vi "AIT 664 - Read Parameters Input VL.vi"(0 "Input VL Parameter File":T1, 5 "Found VL?":bool, 7 "Input VLs":T1[](array[typedef]), 9 "Input VL Configuration File":T1, 11 "error in (no error)":errorcluster) -> (4 "Input VLs out":T1[](array[typedef]), 15 "error out":errorcluster)   [LabVIEW 2013, in "AIT 664 Custom Device.lvlib"]
doc: "Match the parameter file with the configuration file input vls"
uses:
  AIT 664 Custom Device.lvlib
  Controls/664 - XML Input VL.ctl
  Controls/664 - XML Rx Message Port.ctl
  Controls/664 - Sampling Type.ctl
  Controls/664 -Param.ctl
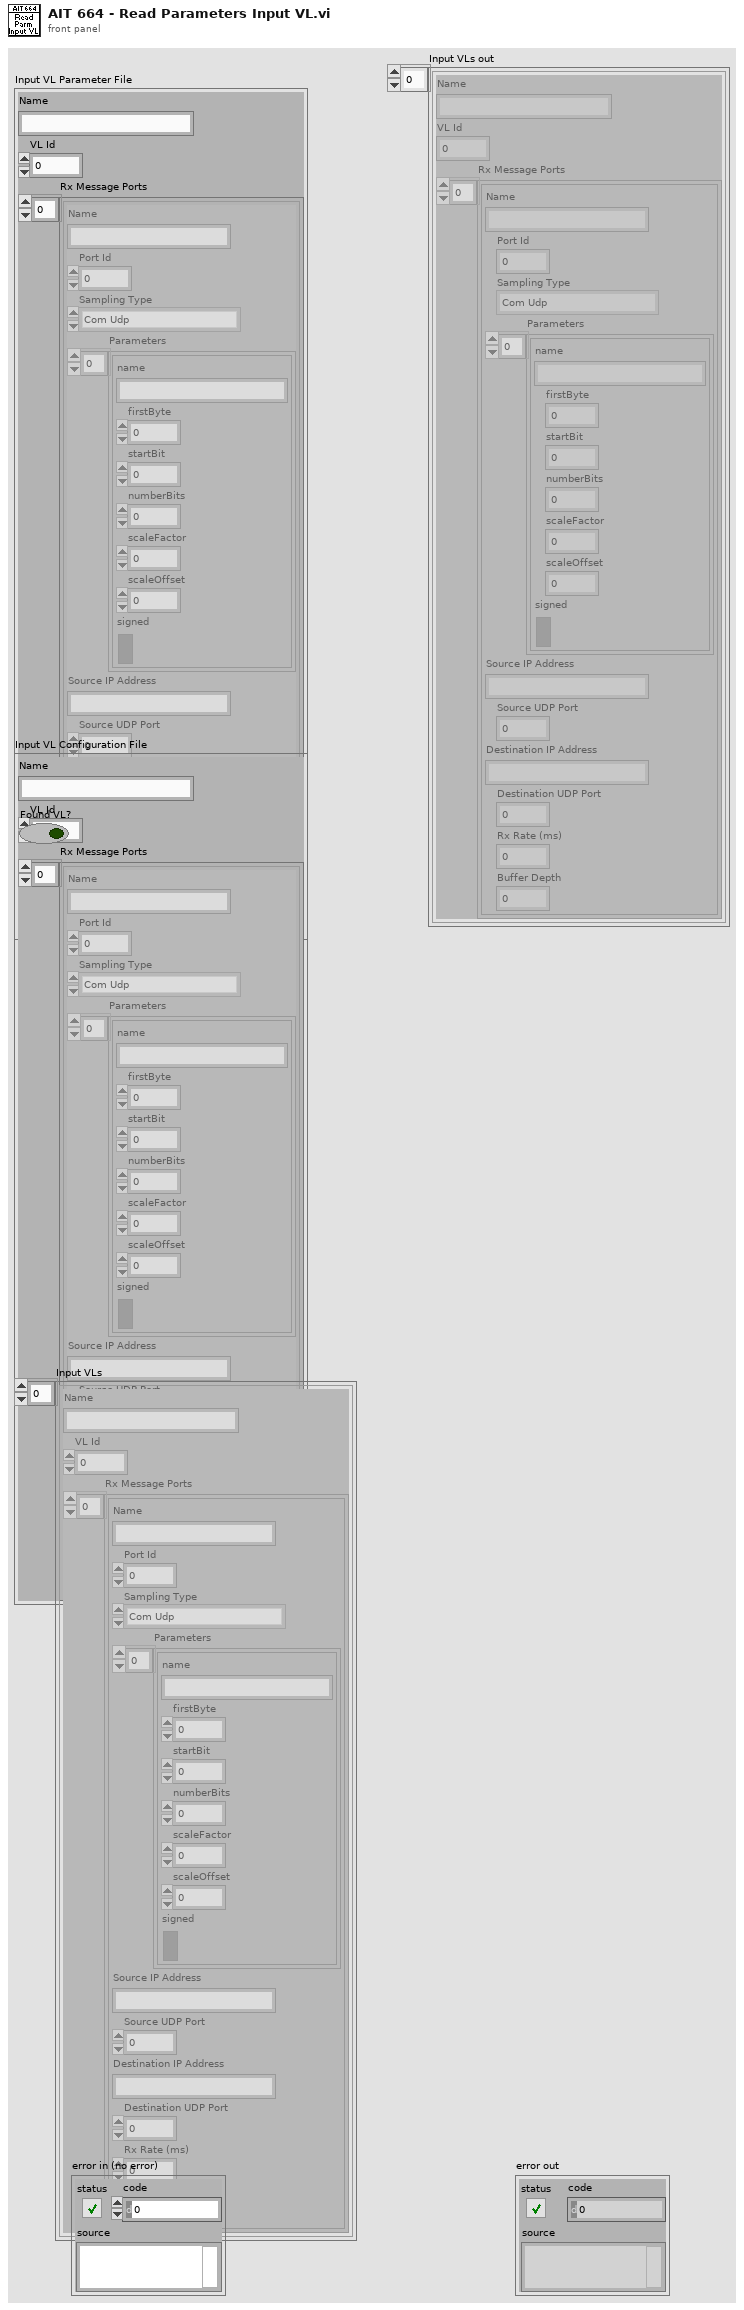
[diagram p1: front panel]
types:
  T1 = typedef "AIT 664 Custom Device.lvlib/664 - XML Input VL.ctl" = cluster{"Name":string, "VL Id":u32, "Rx Message Ports":T2[]}
  T2 = typedef "AIT 664 Custom Device.lvlib/664 - XML Rx Message Port.ctl" = cluster{"Name":string, "Port Id":u32, "Sampling Type":T3, "Parameters":T4[], "Source IP Address":string, "Source UDP Port":u32, "Destination IP Address":string, "Destination UDP Port":u32, "Rx Rate (ms)":u32, "Buffer Depth":u32}
  T3 = typedef "AIT 664 Custom Device.lvlib/664 - Sampling Type.ctl" = enum16{"Com Udp", "Com Udp Queuing", "Sap Udp", "Sap Ip", "Sap Mac", "Unknown"}
  T4 = typedef "AIT 664 Custom Device.lvlib/664 -Param.ctl" = cluster{"name":string, "firstByte":i32, "startBit":i32, "numberBits":i32, "scaleFactor":dbl, "scaleOffset":dbl, "signed":bool}
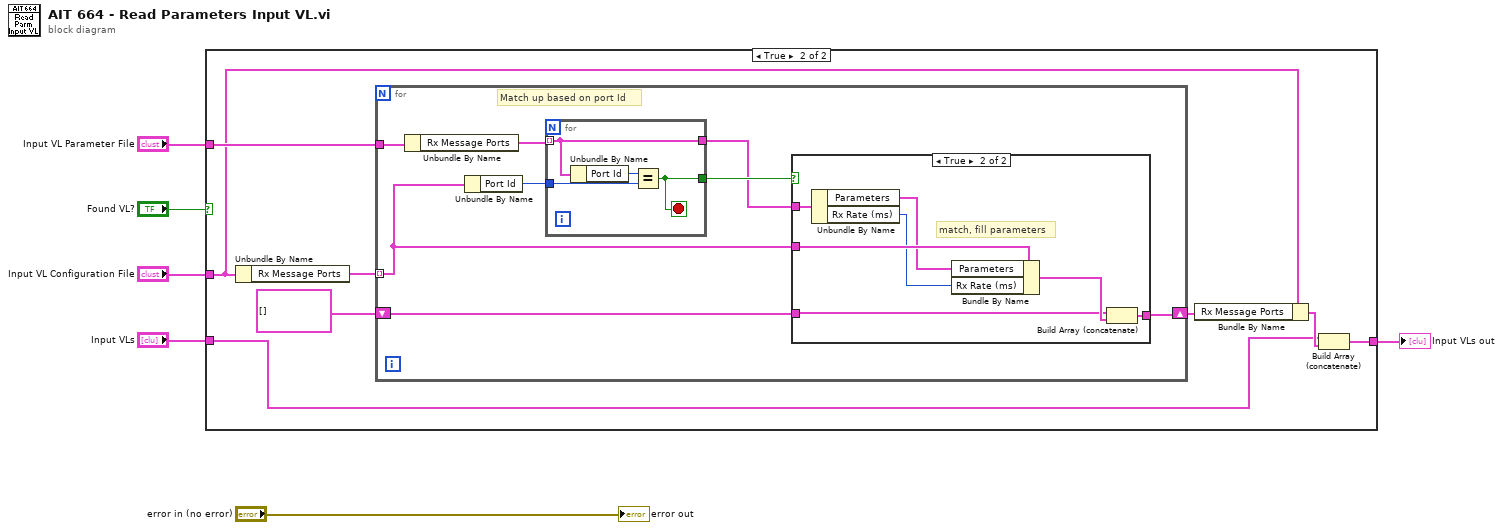
[diagram p0: block diagram]
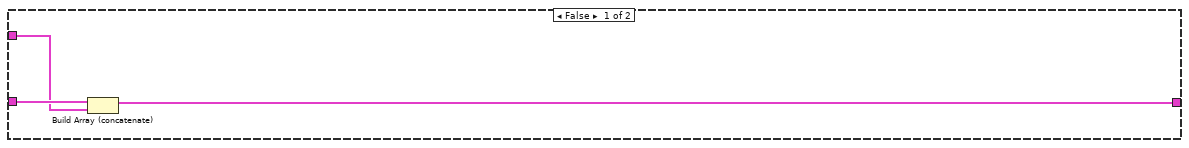
[diagram p2: hidden frame]
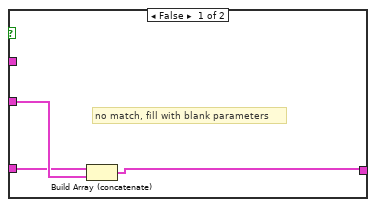
[diagram p3: hidden frame]
diagram:
  n1 = case shown="True" "Found VL?" {
    tunnel: "Input VLs" -> [w9 w10]
    tunnel: [w8 w11] -> w4
    tunnel: "Input VL Configuration File" -> [w7 w14]
    tunnel: "Input VL Parameter File" -> [_ w16]
    frame False {
      n2 = Build Array (concatenate)(w9, w7) -> (w8:T1[])
    }
    frame True {
      n3 = Unbundle By Name(w14) -> ("Rx Message Ports"=w17:T2[])
      n4 = for {
        tunnel: w17 -> [w20] mode=indexing
        tunnel: w16 -> [w25]
        shift-right: [w18] -> w13
        shift-left: T2[] [] -> [w19]
        # "Match up based on port Id"
        n5 = Unbundle By Name(w25) -> ("Rx Message Ports"=w24:T2[])
        n6 = Unbundle By Name(w20) -> ("Port Id"=w23:u32)
        n7 = for {
          tunnel: w24 -> [w36] mode=indexing
          tunnel: w23 -> [w38]
          tunnel: [w37] -> w22
          tunnel: [w36] -> w21
          stop <- w37 stop-if-true
          n8 = Unbundle By Name(w36) -> ("Port Id"=w39:u32)
          n9 = Equal?(x=w39, y=w38) -> (x = y?=w37:bool)
        }
        n10 = case shown="True" w22 {
          tunnel: w21 -> [_ w35]
          tunnel: w20 -> [w28 w34]
          tunnel: w19 -> [w27 w31]
          tunnel: [w26 w30] -> w18
          frame False {
            # "no match, fill with blank parameters"
            n11 = Build Array (concatenate)(w27, w28) -> (w26:T2[])
          }
          frame True {
            # "match, fill parameters"
            n12 = Unbundle By Name(w35) -> ("Parameters"=w33:T4[], "Rx Rate (ms)"=w29:u32)
            n13 = Bundle By Name(cluster=w34, "Parameters"=w33, "Rx Rate (ms)"=w29) -> (w32:T2)
            n14 = Build Array (concatenate)(w31, w32) -> (w30:T2[])
          }
        }
      }
      n15 = Bundle By Name(cluster=w14, "Rx Message Ports"=w13) -> (w12:T1)
      n16 = Build Array (concatenate)(w10, w12) -> (w11:T1[])
    }
  }
  "Input VLs out" <- w4
  "error out" <- "error in (no error)"
